vi "NIDCPower_channel_ganging - Configure Digital Edge Measure Trigger.vi"(8 "error in (no error)":errorcluster, 9 "output terminal":tag, 10 "edge (rising)":T1=1016 items=["Rising"=1016, "Falling"=1017], 11 "Ganged Session in":T2) -> (0 "error out":errorcluster, 3 "Ganged Session out":T2)   [LabVIEW 2021]
uses:
  ctl/NIDCPower_channel_ganging - ctl - channel mode.ctl
  <instrlib>/niDCPower/nidcpower.llb/niDCPower Configure Digital Edge Measure Trigger With Channels.vi
  ctl/NIDCPower_channel_ganging - ctl - ganged config.ctl
  ctl/NIDCPower_channel_ganging - ctl - ganged session.ctl
  <instrlib>/niDCPower/nidcpower.llb/niDCPower Digital Edge - Edge.ctl
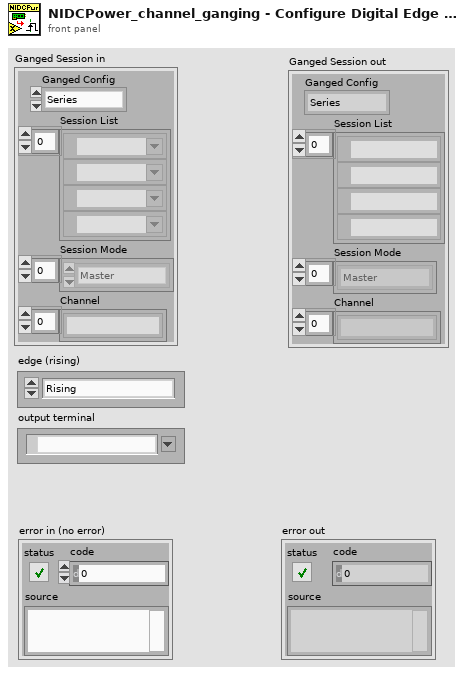
[diagram p1: front panel]
types:
  T1 = typedef "niDCPower Digital Edge - Edge.ctl" = i32
  T2 = typedef "NIDCPower_channel_ganging - ctl - ganged session.ctl" = cluster{"Ganged Config":T3, "Session List":refnum<k15>[], "Session Mode":T4[], "Channel":string[]}
  T3 = typedef "NIDCPower_channel_ganging - ctl - ganged config.ctl" = enum16{"Series", "Parallel", "Manual"}
  T4 = typedef "NIDCPower_channel_ganging - ctl - channel mode.ctl" = enum16{"Master", "Slave", "Slave - Inverted"}
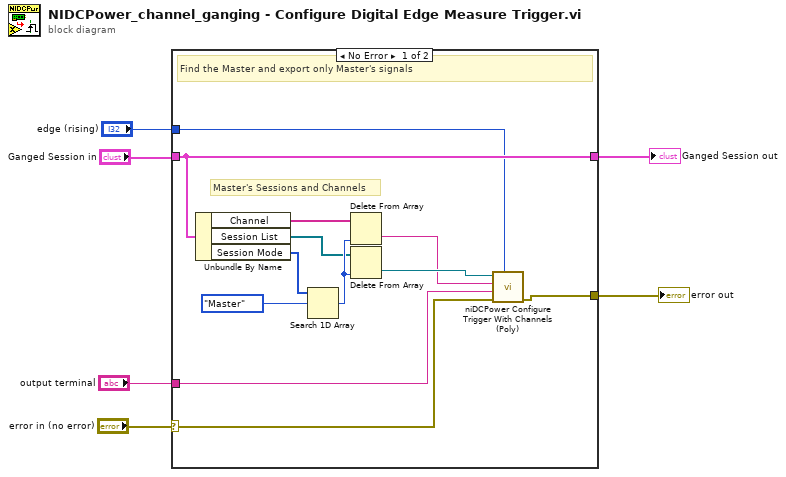
[diagram p0: block diagram]
diagram:
  n1 = case shown="No Error" "error in (no error)" {
    selector: "error in (no error)" -> [w10 w20]
    tunnel: [w8 w20] -> w6
    tunnel: "Ganged Session in" -> [w17 w19]
    tunnel: [w17 w19] -> w4
    tunnel: "output terminal" -> [w9 _]
    tunnel: "edge (rising)" -> [w7 _]
    frame No Error {
      # "Master's Sessions and Channels"
      # "Find the Master and export only Master's signals"
      n2 = Unbundle By Name(w17) -> ("Channel"=w15:string[], "Session List"=w14:refnum<k15>[], "Session Mode"=w13:T4[])
      n3 = Search 1D Array(1D array=w13, element=NIDCPower_channel_ganging_-_ctl_-_channel_mode."Master" ("Channel Mode")) -> (index of element=w16:i32)  [unwired: 1 in]
      n4 = Delete From Array(array=w15, index=w16) -> (deleted portion=w11:string)  [unwired: 1 in, 1 out]
      n5 = Delete From Array(array=w14, index=w16) -> (deleted portion=w12:refnum<k15>)  [unwired: 1 in, 1 out]
      n6 = call-poly <instrlib>:"niDCPower Configure Trigger With Channels (Poly).vi"("edge (rising)"=w7, "error in (no error)"=w10, "input terminal"=w9, "channel name"=w11, "instrument handle"=w12) -> ("error out"=w8:errorcluster)  [unwired: 5 in, 1 out]
    }
    frame Error {
    }
  }
  "error out" <- w6
  "Ganged Session out" <- w4
